vi "niRFUtil FTW Brickwall Filter (complex wfm).vi"(0 "Waveform In (V)":T1 {"y" format="%.2f"; "dx" format="%^.2e"; "x0" format="%^.2e"}, 5 "Center Frequency (Hz)":dbl format="%^.6e", 7 "Bandwidth (Hz)":dbl=1000000.0 format="%^.6e") -> (4 "Waveform Out (V)":T1 {"y" format="%.2f"; "dx" format="%^.2e"; "x0" format="%^.2e"})   [LabVIEW 2015, in "niRFUtil.lvlib"]
doc: "(c) Copyright 2006, National Instruments, Inc. This VI may not be duplicated, sold, or distributed without written consent from National Instruments."
uses:
  niRFUtil.lvlib
  Includes/niRFUtil INC Complex Waveform.ctl
  Includes/niRFUtil INC Complex Array.ctl
  niRFUtil FTW FFT (complex wfm).vi
  Measurements/niRFUtil MEAS Waveform Statistics (complex wfm).vi
  Waveform Manipulation/niRFUtil WFM Multiply Waveforms (complex wfm).vi
  niRFUtil FTW IFFT (complex wfm).vi
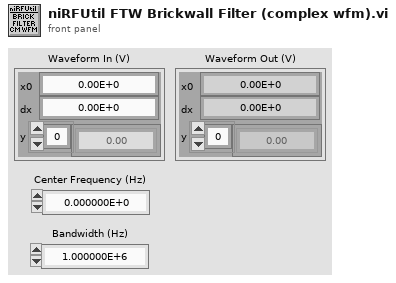
[diagram p1: front panel]
types:
  T1 = typedef "niRFUtil.lvlib/niRFUtil INC Complex Waveform.ctl" = cluster{"x0":dbl, "dx":dbl, "y":T2}
  T2 = typedef "niRFUtil.lvlib/niRFUtil INC Complex Array.ctl" = csg[]
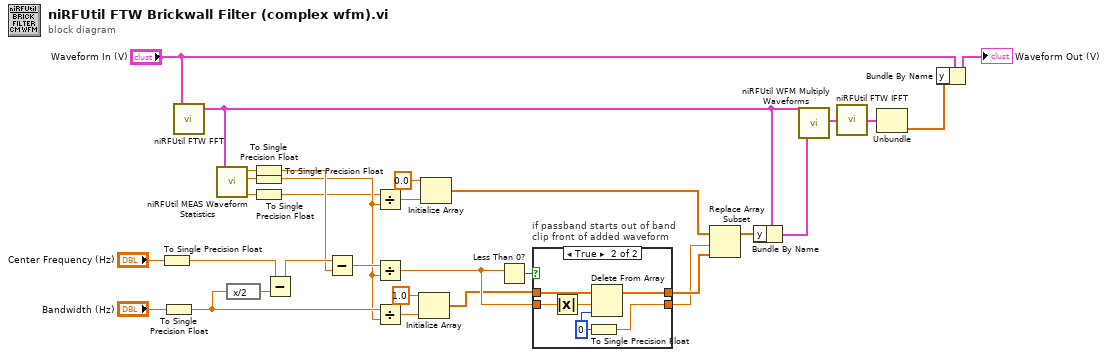
[diagram p0: block diagram]
diagram:
  n1 = To Single Precision Float(number="Center Frequency (Hz)") -> (single precision float=w10:sgl)
  n2 = To Single Precision Float(number="Bandwidth (Hz)") -> (single precision float=w9:sgl)
  n3 = call-poly "niRFUtil FTW FFT.vi"("Waveform In (V)"="Waveform In (V)") -> ("Waveform Out (V)"=w19:T1)  [unwired: 2 in, 2 out]
  n4 = call-poly "niRFUtil MEAS Waveform Statistics.vi"("Waveform In"=w19) -> ("Start"=w28:dbl, "Interval"=w23:dbl, "Duration"=w31:dbl)  [unwired: 5 out]
  n5 = expression code="x/2"(w9) -> (w25:sgl)
  n6 = To Single Precision Float(number=w28) -> (single precision float=w8:sgl)
  n7 = To Single Precision Float(number=w23) -> (single precision float=w7:sgl)
  n8 = To Single Precision Float(number=w31) -> (single precision float=w6:sgl)
  n9 = Subtract(x=w10, y=w25) -> (x-y=w24:sgl)
  n10 = Subtract(x=w24, y=w8) -> (x-y=w27:sgl)
  n11 = Divide(x=w6, y=w7) -> (x/y=w30:sgl)
  n12 = Divide(x=w27, y=w7) -> (x/y=w13:sgl)
  n13 = Divide(x=w9, y=w7) -> (x/y=w21:sgl)
  n14 = Initialize Array(sgl 1.0 ("element"), w21) -> (w12:sgl[])
  n15 = Initialize Array(sgl 0.0 ("element"), w30) -> (w26:sgl[])
  n16 = Less Than 0?(x=w13) -> (x < 0?=w15:bool)
  n17 = case "if passband starts out of band\nclip front of added waveform" shown="True" w15 {
    tunnel: w12 -> [w33 w35]
    tunnel: [w33 w39] -> w14
    tunnel: w13 -> [w32 w36]
    tunnel: [w32 w34] -> w11
    frame False {
    }
    frame True {
      w38 = 0 ("index")
      n18 = Absolute Value(x=w36) -> (abs(x)=w37:sgl)
      n19 = To Single Precision Float(number=w38) -> (single precision float=w34:sgl)
      n20 = Delete From Array(array=w35, length=w37, index=w38) -> (array with subset deleted=w39:sgl[])  [unwired: 1 out]
    }
  }
  n21 = Replace Array Subset(array=w26, new element=w14, index=w11) -> (w20:sgl[])
  n22 = Bundle By Name(cluster=w19, "y"=w20) -> (w18:T1)
  n23 = call-poly "niRFUtil WFM Multiply Waveforms.vi"("Waveform 2 In"=w18, "Waveform 1 In"=w19) -> ("Waveform Out"=w17:T1)  [unwired: 1 out]
  n24 = call-poly "niRFUtil FTW IFFT.vi"("Waveform In (V)"=w17) -> ("Waveform Out (V)"=w16:T1)
  n25 = Unbundle(w16) -> ("y"=w1:T2)  [unwired: 2 out]
  n26 = Bundle By Name(cluster="Waveform In (V)", "y"=w1) -> (→"Waveform Out (V)":T1)
